vi "error_handler.vi"(5 "session in":T1={"VISA resource out"="COM12", "error out"={"status"=FALSE, "code"=0, "source"=""}}) -> (0 "error out":errorcluster, 1 "error?":bool, 2 "session out":T1={"VISA resource out"="COM12", "error out"={"status"=FALSE, "code"=0, "source"=""}})   [LabVIEW 2010]
uses:
  error_messages_global.vi
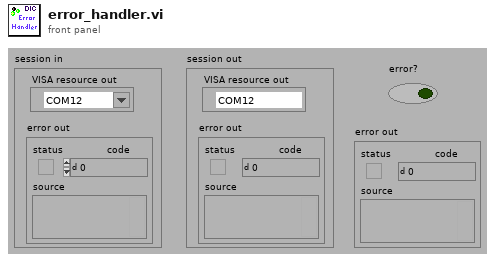
[diagram p1: front panel]
types:
  T1 = cluster{"VISA resource out":refnum<visa-resource-name>, "error out":errorcluster}
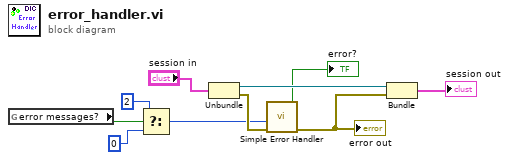
[diagram p0: block diagram]
diagram:
  n1 = global read "error_messages_global.vi" "error messages?"() -> (w3:bool)
  n2 = Select(t=2, s=w3, f=0) -> (s? t:f=w2:i32)
  n3 = Unbundle("session in") -> ("VISA resource out"=w8:refnum<visa-resource-name>, "error out"=w7:errorcluster)
  n4 = call <vilib>:"Simple Error Handler.vi"("type of dialog (OK msg:1)"=w2, "error in (no error)"=w7) -> ("error?"=→"error?":bool, "error out"=w1:errorcluster)  [unwired: 3 in, 3 out]
  "error out" <- w1
  n5 = Bundle("VISA resource out"=w8, "error out"=w1) -> (→"session out":T1)  [unwired: 1 in]
